vi "Dispose Fiducial Images.vi"(5 "Archive":bool, 7 "Dispose":bool, 8 "error in":errorcluster, 11 "Potting Procedure in":refnum<class "Potting Procedure.lvclass">) -> (0 "error out":errorcluster, 3 "Potting Procedure out":refnum<class "Potting Procedure.lvclass">)   [LabVIEW 2017, in "Potting Procedure.lvclass"]
uses:
  Potting Procedure.lvclass
  Shared Components/Gantry Class/Gantry Class.lvclass
  Shared Components/Config Manager Class/Config Manager Class.lvclass
  Shared Components/Vec3d Class/Vec3d Class.lvclass
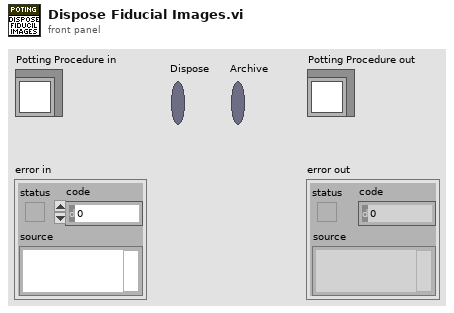
[diagram p1: front panel]
types:
  T1 = typedef "Fiducial Image.ctl" = cluster{"Fiducial Image":T2, "Selected Fiducial":T4, "fiducial name":string}
  T2 = typedef "Physical Image.ctl" = cluster{"Image Position":refnum<class "Vec3d Class.lvclass">, "Image Reference":T3, "Field of View":cluster{"x(mm)":dbl, "y(mm)":dbl}}
  T3 = typedef "IMAQ Image.ctl" = refnum<image>
  T4 = typedef "Fiducial with Source.ctl" = cluster{"Fiducial Image Coordinate":refnum<class "Vec3d Class.lvclass">, "Fiducial Source":enum16{"Pattern Recognition", "User", "Error", "Default"}}
  T5 = cluster{"Fiducials-HDI":T1[], "Fiducials-BBM":T1[], "Chuck":i32, "Slot":i32}[]
  T6 = cluster{"Fiducials-HDI":T1[], "Fiducials-BBM":T1[], "Chuck":i32, "Slot":i32}
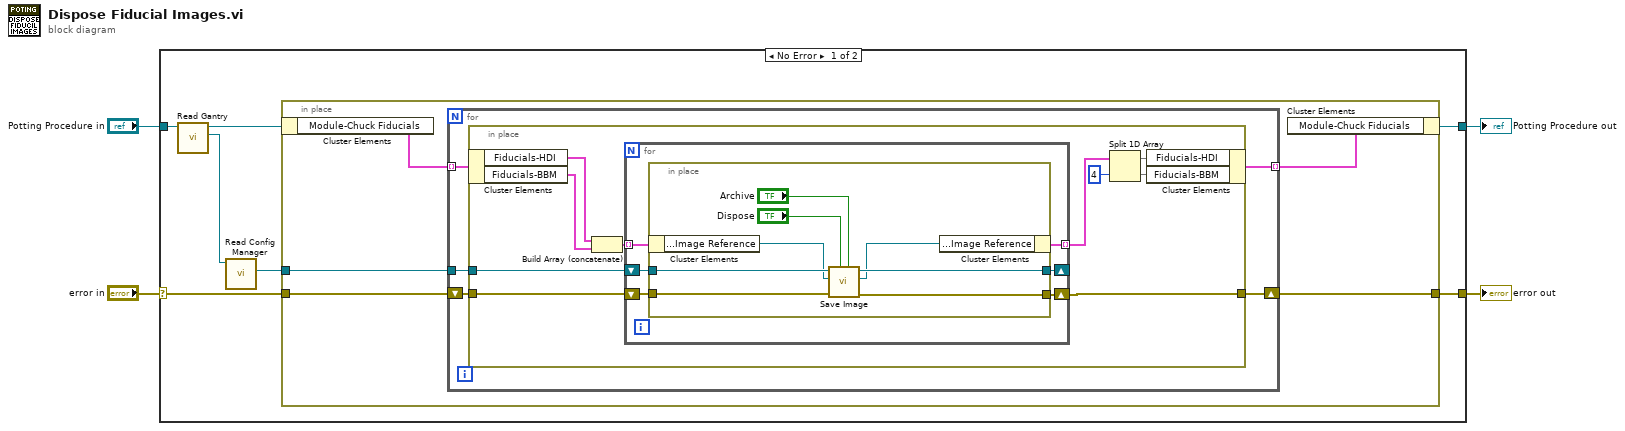
[diagram p0: block diagram]
diagram:
  n1 = case shown="No Error" "error in" {
    selector: "error in" -> [w11 w47]
    tunnel: [w10 w47] -> w3
    tunnel: [w9 w46] -> w1
    tunnel: "Potting Procedure in" -> [w8 w46]
    frame No Error {
      n2 = call-dynamic "Read Gantry.vi"("Potting Procedure in"=w8) -> ("Gantry"=w6:refnum<class "Gantry Class.lvclass">, "Potting Procedure out"=w7:refnum<class "Potting Procedure.lvclass">)  [unwired: 8 in, 1 out]
      n3 = call-dynamic "Read Config Manager.vi"("Gantry in"=w6) -> ("Config Manager"=w5:refnum<class "Config Manager Class.lvclass">)  [unwired: 8 in, 2 out]
      n4 = in-place {
        in-place-border: w11 -> [w16]
        in-place-border: [w15] -> w10
        in-place-border: w5 -> [w12]
        n5 = in-place-cluster #1(w7) -> ("Module-Chuck Fiducials"=w14:T5)
        n6 = for {
          tunnel: w14 -> [w21] mode=indexing
          tunnel: [w20] -> w13 mode=indexing
          shift-right: [w18] -> w15
          shift-left: w16 -> [w19]
          tunnel: w12 -> [w17]
          n7 = in-place {
            in-place-border: w19 -> [w27]
            in-place-border: [w26] -> w18
            in-place-border: w17 -> [w28]
            n8 = in-place-cluster #2(w21) -> ("Fiducials-HDI"=w31:T1[], "Fiducials-BBM"=w30:T1[])
            n9 = Build Array (concatenate)(w31, w30) -> (w29:T1[])
            n10 = for {
              tunnel: w29 -> [w37] mode=indexing
              tunnel: [w36] -> w25 mode=indexing
              shift-right: [w34] -> _
              shift-left: w28 -> [w35]
              shift-right: [w32] -> w26
              shift-left: w27 -> [w33]
              n11 = in-place {
                in-place-border: w35 -> [w45]
                in-place-border: [w44] -> w34
                in-place-border: w33 -> [w39]
                in-place-border: [w38] -> w32
                n12 = in-place-cluster #3(w37) -> ("Fiducial Image.Image Reference"=w41:T3)
                n13 = call "Save Image.vi"("Archive"="Archive", "Dispose"="Dispose", "error in"=w39, "Image in"=w41, "Config Manager in"=w45) -> ("error out"=w38:errorcluster, "Image out"=w40:T3, "Config Manager out"=w44:refnum<class "Config Manager Class.lvclass">)  [unwired: 4 in]
                n14 = in-place-cluster #3("Fiducial Image.Image Reference"=w40) -> (w36:T1)
              }
            }
            n15 = Split 1D Array(array=w25, index=4) -> (first subarray=w23:T1[], second subarray=w22:T1[])
            n16 = in-place-cluster #2("Fiducials-HDI"=w23, "Fiducials-BBM"=w22) -> (w20:T6)
          }
        }
        n17 = in-place-cluster #1("Module-Chuck Fiducials"=w13) -> (w9:refnum<class "Potting Procedure.lvclass">)
      }
    }
    frame Error {
    }
  }
  "error out" <- w3
  "Potting Procedure out" <- w1
